vi "Check_Timer.vi"(8 "error in (no error)":errorcluster, 10 "Target Duration":dbl, 11 "Start Timestamp":u32) -> (0 "error out":errorcluster, 3 "Done?":bool)   [LabVIEW 2026]
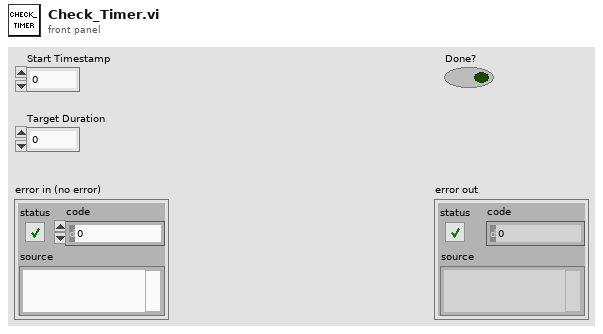
[diagram p1: front panel]
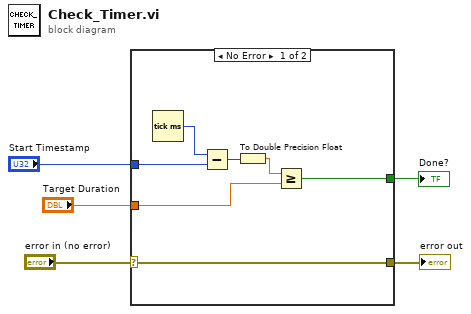
[diagram p0: block diagram]
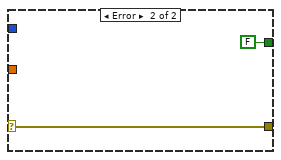
[diagram p2: hidden frame]
diagram:
  n1 = case shown="No Error" "error in (no error)" {
    selector: "error in (no error)" -> [w6 w14]
    tunnel: "Start Timestamp" -> [w12 _]
    tunnel: [w11 FALSE] -> w4
    tunnel: "Target Duration" -> [w8 _]
    tunnel: [w6 w14] -> w1
    frame No Error {
      n2 = Tick Count (ms)() -> (millisecond timer value=w7:u32)
      n3 = Subtract(x=w7, y=w12) -> (x-y=w10:u32)
      n4 = To Double Precision Float(number=w10) -> (double precision float=w9:dbl)
      n5 = Greater Or Equal?(x=w9, y=w8) -> (x >= y?=w11:bool)
    }
    frame Error {
    }
  }
  "Done?" <- w4
  "error out" <- w1
